vi "Start Command.vi"(8 "error in (no error)":errorcluster, 9 "Command Name":string, 10 "Robot Actors.lvlib:Command.lvlib:Command.lvclass":refnum<class "Command.lvclass">, 11 "System Actor in":refnum<class "System Actor.lvclass">) -> (0 "error out":errorcluster, 3 "System Actor out":refnum<class "System Actor.lvclass">)   [LabVIEW 2013, in "Robot Actors.lvlib" / "System Actor.lvlib" / "System Actor.lvclass"]
uses:
  System Actor.lvclass
  Command/Command Class/Command.lvclass
  Command Processor/Command Processor Messages/Start Command Msg/Start Command Msg.lvclass/Start Command Msg.ctl
  <vilib>/ActorFramework/Message Enqueuer/Message Enqueuer.lvclass/Message Enqueuer.ctl
  <vilib>/ActorFramework/Message Enqueuer/Enqueue.vi
  <vilib>/ActorFramework/Message Priority Queue/Priority Enqueue.vi
  Command Processor/Command Processor Messages/Start Command Msg/Start Command Msg.lvclass
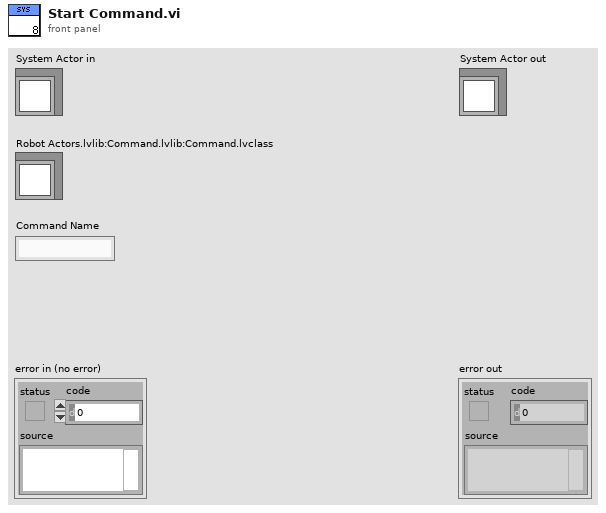
[diagram p1: front panel]
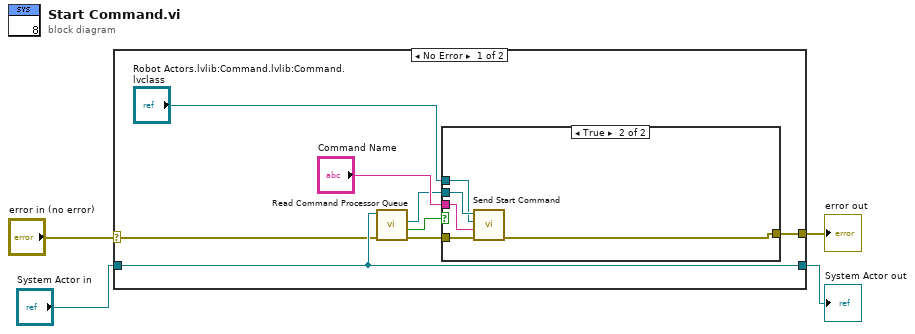
[diagram p0: block diagram]
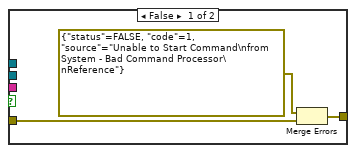
[diagram p2: hidden frame]
diagram:
  n1 = case shown="No Error" "error in (no error)" {
    selector: "error in (no error)" -> [w7 w22]
    tunnel: [w5 w22] -> w3
    tunnel: [w12 w21] -> w1
    tunnel: "System Actor in" -> [w12 w21]
    frame No Error {
      n2 = call-dynamic "Read Command Processor Queue.vi"("error in (no error)"=w7, "System Actor in"=w12) -> ("error out"=w6:errorcluster, "Is Valide Queue?"=w11:bool, "Actor Framework:Message Enqueuer"=w9:refnum<class "Message Enqueuer.lvclass">)  [unwired: 6 in, 1 out]
      n3 = case shown="True" w11 {
        tunnel: "Command Name" -> [_ w20]
        tunnel: w9 -> [_ w19]
        tunnel: "Robot Actors.lvlib:Command.lvlib:Command.lvclass" -> [_ w18]
        tunnel: w6 -> [w15 w17]
        tunnel: [w14 w16] -> w5
        frame False {
          n4 = Merge Errors(errorcluster {"status"=FALSE, "code"=1, "source"="Unable to Start Command\nfrom System - Bad Command Processor\nReference"} ("error in"), w15) -> (w14:errorcluster)
        }
        frame True {
          n5 = call "Send Start Command.vi"("error in (no error)"=w17, "Command Name"=w20, "Robot Actors.lvlib:Command.lvlib:Command.lvclass"=w18, "Message Enqueuer"=w19) -> ("error out"=w16:errorcluster)  [unwired: 6 in, 1 out]
        }
      }
    }
    frame Error {
    }
  }
  "error out" <- w3
  "System Actor out" <- w1
